vi "boxdata.vi"(7 "Box Width":dbl=10.0 format="%.2f", 10 "Plot #":u32, 11 "Raw Data":dbl[](array[numeric]) format="%.2f") -> (2 "XY Graph":cluster{dbl[], dbl[]}[](graph))   [LabVIEW 2021, in "statistics.lvlib"]
uses:
  statistics.lvlib
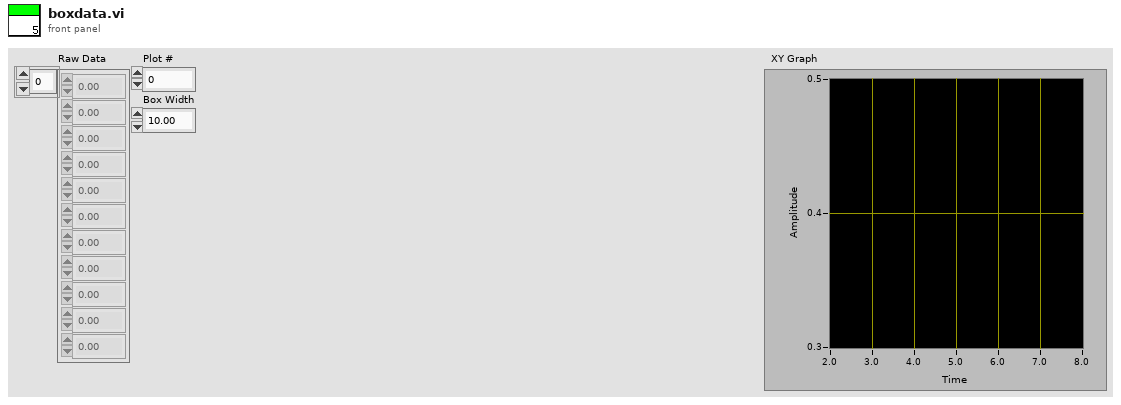
[diagram p1: front panel]
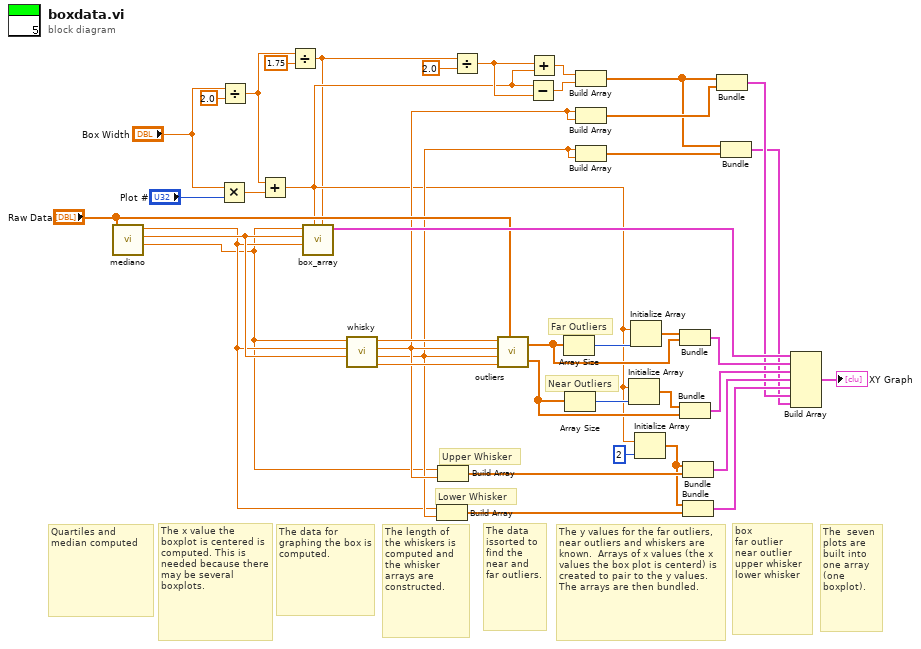
[diagram p0: block diagram]
diagram:
  # "box\nfar outlier\nnear outlier\nupper whisker\nlower whisker"
  # "The data issorted to find the near and far outliers."
  # "The length of the whiskers is computed and the whisker arrays are constructed."
  # "The data for graphing the box is computed."
  # "The x value the boxplot is centered is computed. This is needed because there may be several boxplots."
  # "Quartiles and median computed"
  # "The  seven plots are built into one array (one boxplot)."
  # "Near Outliers"
  # "Far Outliers"
  # "The y values for the far outliers, near outliers and whiskers are known.  Arrays of x values (the x values the box plot is centerd) is created to pair to the y values.  The arrays are then bundled."
  # "Lower Whisker"
  # "Upper Whisker"
  n1 = call "mediano.vi"("data"="Raw Data") -> ("Q3"=w1:dbl, "median"=w22:dbl, "Q1"=w2:dbl)  [unwired: 8 in]
  n2 = Multiply(x="Box Width", y="Plot #") -> (x*y=w21:dbl)
  n3 = Divide(x="Box Width", y=2.0 ("x")) -> (x/y=w4:dbl)
  n4 = Add(x=w4, y=w21) -> (x+y=w8:dbl)
  n5 = Divide(x=w4, y=1.75 ("x")) -> (x/y=w3:dbl)
  n6 = call "box_array.vi"("Box Width"=w3, "X position"=w8, "Lower Quartile (LQ)"=w2, "Median"=w22, "Upper Quartile (UQ)"=w1) -> ("XY Graph"=w29:cluster{dbl[], dbl[]})  [unwired: 6 in]
  n7 = call "whisky.vi"("Median"=w22, "Lower Quartile (LQ)"=w2, "Upper Quartile (UQ)"=w1) -> ("L2"=w30:dbl, "L1"=w9:dbl, "U1"=w18:dbl, "U2"=w31:dbl)  [unwired: 1 in]
  n8 = Build Array(w2, w9) -> (w33:dbl[])
  n9 = Build Array(w1, w18) -> (w34:dbl[])
  n10 = Divide(x=w3, y=2.0) -> (x/y=w14:dbl)
  n11 = call "outliers.vi"("U2"=w31, "U1"=w18, "L1"=w9, "L2"=w30, "Raw Data"="Raw Data") -> ("Far Outliers"=w36:dbl[], "Near Outliers"=w37:dbl[])
  n12 = Subtract(x=w8, y=w14) -> (x-y=w15:dbl)
  n13 = Add(x=w14, y=w8) -> (x+y=w16:dbl)
  n14 = Array Size(array=w36) -> (size(s)=w41:i32)
  n15 = Array Size(array=w37) -> (size(s)=w40:i32)
  n16 = Build Array(w16, w15) -> (w11:dbl[])
  n17 = Build Array(w18, w18) -> (w12:dbl[])
  n18 = Build Array(w9, w9) -> (w10:dbl[])
  n19 = Initialize Array(w8, w40) -> (w38:dbl[])
  n20 = Initialize Array(w8, w41) -> (w39:dbl[])
  n21 = Initialize Array(w8, 2 ("dimension size")) -> (w32:dbl[])
  n22 = Bundle(w39, "Far Outliers"=w36) -> (w28:cluster{dbl[], "Far Outliers":dbl[]})  [unwired: 1 out]
  n23 = Bundle(w38, "Near Outliers"=w37) -> (w27:cluster{dbl[], "Near Outliers":dbl[]})  [unwired: 1 out]
  n24 = Bundle(w32, w34) -> (w26:cluster{dbl[], dbl[]})  [unwired: 1 out]
  n25 = Bundle(w32, w33) -> (w25:cluster{dbl[], dbl[]})  [unwired: 1 out]
  n26 = Bundle(w11, w12) -> (w20:cluster{dbl[], dbl[]})  [unwired: 1 out]
  n27 = Bundle(w11, w10) -> (w13:cluster{dbl[], dbl[]})  [unwired: 1 out]
  n28 = Build Array(w29, w28, w27, w26, w25, w20, w13) -> (→"XY Graph":cluster{dbl[], "Near Outliers":dbl[]}[])
